vi "VI Tree.vi"   [LabVIEW 2010, in "Agilent E363X Series.lvlib"]
doc: "This is the instrument driver for the Agilent E363xA. The VI Tree displays all the user-callable VIs of the instrument driver in an organized table."
uses:
  <instrlib>/Agilent E363X Series/Agilent E363X Series.lvlib
panel:
  # "(c) 2008 National Instruments.  ALL RIGHTS RESERVED."
  # "SEE DIAGRAM\nFOR VI TREE."
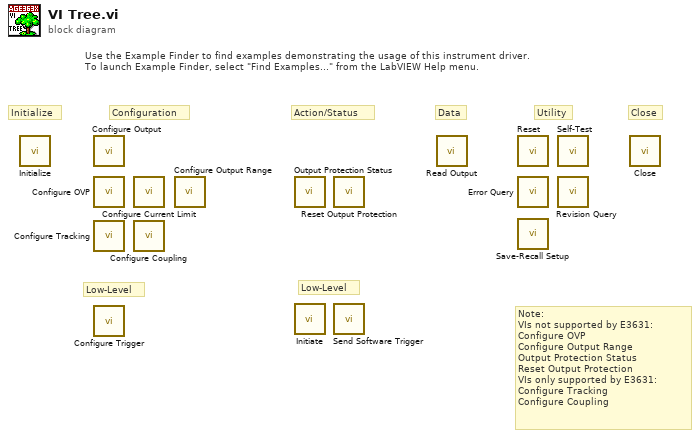
[diagram p0: block diagram]
diagram:
  # "Note:\nVIs not supported by E3631:\nConfigure OVP\nConfigure Output Range\nOutput Protection Status\nReset Output Protection\nVIs only supported by E3631:\nConfigure Tracking\nConfigure Coupling"
  # "Low-Level"
  # "Low-Level"
  # "Use the Example Finder to find examples demonstrating the usage of this instrument driver.\nTo launch Example Finder, select \"Find Examples...\" from the LabVIEW Help menu."
  # "Configuration"
  # "Utility"
  # "Data"
  # "Action/Status"
  # "Close"
  # "Initialize"
  n1 = call <instrlib>:"Initialize.vi"() -> ()  [unwired: 10 in, 2 out]
  n2 = call <instrlib>:"Configure Output.vi"() -> ()  [unwired: 10 in, 2 out]
  n3 = call <instrlib>:"Configure OVP.vi"() -> ()  [unwired: 10 in, 2 out]
  n4 = call <instrlib>:"Configure Tracking.vi"() -> ()  [unwired: 10 in, 2 out]
  n5 = call <instrlib>:"Configure Trigger.vi"() -> ()  [unwired: 10 in, 2 out]
  n6 = call <instrlib>:"Configure Current Limit.vi"() -> ()  [unwired: 10 in, 2 out]
  n7 = call <instrlib>:"Configure Coupling.vi"() -> ()  [unwired: 10 in, 2 out]
  n8 = call <instrlib>:"Configure Output Range.vi"() -> ()  [unwired: 10 in, 2 out]
  n9 = call <instrlib>:"Output Protection Status.vi"() -> ()  [unwired: 8 in, 4 out]
  n10 = call <instrlib>:"Initiate.vi"() -> ()  [unwired: 10 in, 2 out]
  n11 = call <instrlib>:"Reset Output Protection.vi"() -> ()  [unwired: 10 in, 2 out]
  n12 = call <instrlib>:"Send Software Trigger.vi"() -> ()  [unwired: 10 in, 2 out]
  n13 = call <instrlib>:"Read Output.vi"() -> ()  [unwired: 8 in, 4 out]
  n14 = call <instrlib>:"Reset.vi"() -> ()  [unwired: 10 in, 2 out]
  n15 = call <instrlib>:"Error Query.vi"() -> ()  [unwired: 8 in, 4 out]
  n16 = call <instrlib>:"Save-Recall Setup.vi"() -> ()  [unwired: 10 in, 2 out]
  n17 = call <instrlib>:"Self-Test.vi"() -> ()  [unwired: 8 in, 4 out]
  n18 = call <instrlib>:"Revision Query.vi"() -> ()  [unwired: 8 in, 4 out]
  n19 = call <instrlib>:"Close.vi"() -> ()  [unwired: 11 in, 1 out]
